vi "ReadCSVFile.vi"() -> ()   [LabVIEW 2018]
uses:
  <vilib>/Utility/file.llb/Read Delimited Spreadsheet (string).vi
panel:
  out "Table":string[][](table)
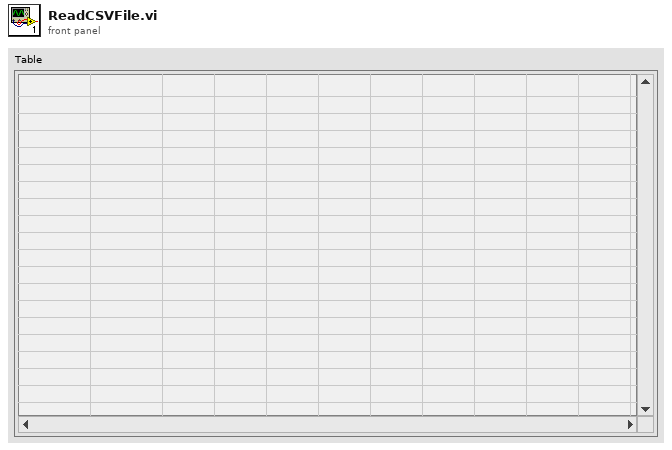
[diagram p1: front panel]
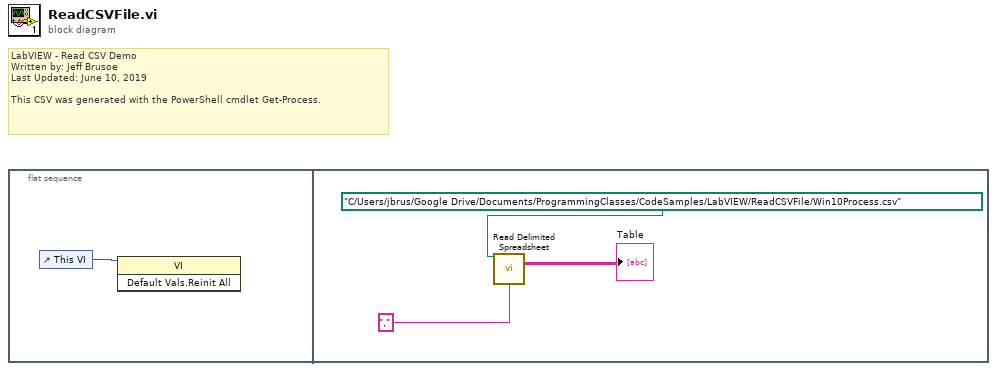
[diagram p0: block diagram]
diagram:
  # "LabVIEW - Read CSV Demo\nWritten by: Jeff Brusoe\nLast Updated: June 10, 2019\n\nThis CSV was generated with the PowerShell cmdlet Get-Process."
  n1 = flat-sequence {
    frame #0 {
      n2 = control-ref of="This VI"() -> (w1:refnum<vi>)
      n3 = invoke class="VI" method="Default Vals.Reinit All"(reference=w1) -> ()  [unwired: 2 in, 3 out]
    }
    frame #1 {
      n4 = call-poly <vilib>:"Read Delimited Spreadsheet.vi"("file path (dialog if empty)"=path "C:/Users/jbrus/Google Drive/Documents/ProgrammingClasses/CodeSamples/LabVIEW/ReadCSVFile/Win10Process.csv", "delimiter (\\t)"=",") -> ("all rows"=→"Table":string[][])  [unwired: 8 in, 5 out]
    }
  }
